vi "Catch Nested Value Update.vi"(8 "error in (no error)":errorcluster, 10 "Nested Value Update Msg":refnum<class "Nested Value Update Msg.lvclass">, 11 "ViewModel In":refnum<class "Test Executive Builder ViewModel.lvclass">) -> (0 "error out":errorcluster, 3 "ViewModel Out":refnum<class "Test Executive Builder ViewModel.lvclass">)   [LabVIEW 2017, in "Test Executive Builder ViewModel.lvclass"]
doc: "<License>\nCopyright © 2017 Composed Systems, LLC | All rights reserved\nwww.composed.io\n\nAuthor: Ethan Stern <ethan.stern@composed.io>\n\nThis software is provided \"AS IS\" WITHOUT WARRANTIES, either express or implied, AND IS FOR EDUCATIONAL PURPOSES ONLY.\n</License>"
uses:
  Test Executive Builder ViewModel.lvclass
  <vilib>/gpm_packages/@cs/mva-viewable/Source/IViewModel/IViewModel/IViewModel.lvclass
  <vilib>/gpm_packages/@cs/mva-viewable/Source/IViewable/IViewable Messages/Catch Nested Value Change Msg/Nested Value Update Msg.lvclass
  C:/Users/jonmc/Documents/Git/Test Executive Builder/gpm_packages/@cs/mva-viewable/Source/IViewModel/IViewModel/IViewModel.lvclass
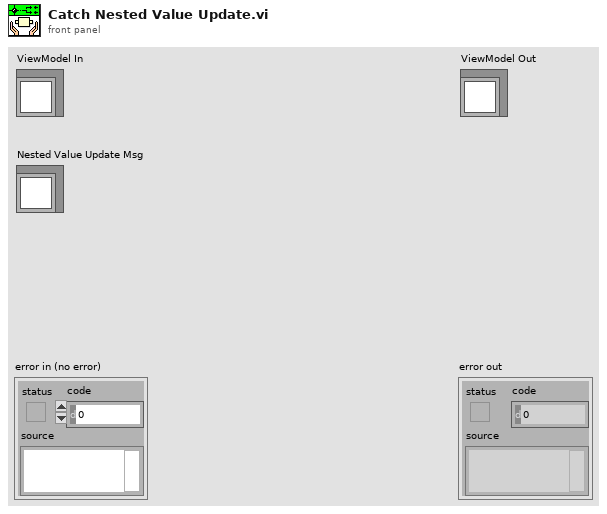
[diagram p1: front panel]
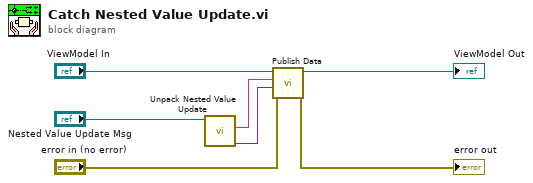
[diagram p0: block diagram]
diagram:
  n1 = call <vilib>:"Unpack Nested Value Update.vi"("Nested Value Update Msg"="Nested Value Update Msg") -> ("Value"=w1:variant, "Datum Name"=w2:string)  [unwired: 8 in, 1 out]
  n2 = call <vilib>:"Publish Data.vi"("error in (no error)"="error in (no error)", "Data to Publish"=w1, "Datum Name"=w2, "IViewModel In"="ViewModel In") -> ("error out"=→"error out":errorcluster, "IViewModel Out"=→"ViewModel Out":refnum<class "Test Executive Builder ViewModel.lvclass">)  [unwired: 6 in]
